vi "AlliGator Get Python Plugin Function Parameters String.vi"(8 "error in (no error)":errorcluster, 10 "Function Parameters":T1[](array[typedef]), 11 "Function Display Name":string) -> (0 "error out":errorcluster, 2 "Function Parameters JSON String":string, 3 "Parameter Names Not Found":string[](array[string]))   [LabVIEW 2021, in "AlliGator Python Plugins.lvlib"]
doc: "Gets requested parameter names from the python function description, opens up a dialog window to allow the user to enter the required parameters, and builds a JSON string to pass those parameters (names and values) to the python function."
uses:
  AlliGator Python Plugins.lvlib
  AlliGator Python Function Parameter Definition.ctl
  AlliGator Variables List.ctl
  d4008f8b-8ee3-446b-8e9c-2fee3dc7eda3.vi
  <userlib>/_OpenG.lib/string/string.llb/To Proper Case (String)__ogtk.vi
  <vilib>/JDP Science/JSONtext/Variant to JSON Text.vi
  <vilib>/JDP Science/JSONtext/support/Format JSON Object.vi
  <vilib>/JDP Science/JSONtext/LVClass Serializer/JSONtext LVClass Serializer.lvclass
  AlliGator Settings.lvlib
  AlliGator Globals, Variables & Constants.lvlib
  <vilib>/JDP Science/JSONtext/JSONtext.lvlib
  <userlib>/_OpenG.lib/string/string.llb/openg_string.lvlib
panel:
  # "see the AlliGator License on the block diagram (Ctrl+E or Window:Show Block Diagram)"
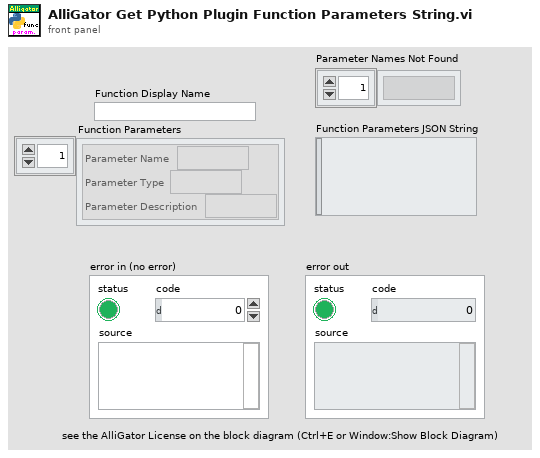
[diagram p1: front panel]
types:
  T1 = typedef "AlliGator Python Plugins.lvlib/AlliGator Python Function Parameter Definition.ctl" = cluster{"Parameter Name":string, "Parameter Type":string, "Parameter Description":string}
  T2 = typedef "AlliGator Globals, Variables & Constants.lvlib/AlliGator Variables List.ctl" = enum16{"---- GUI ----", "Initialization Status", "State Indicators Refnum", "Original AlliGator Menu Items", "Current Action Loop State", "Script in progress", "Playback", "Loop Playback", "Search ROI Used", "Search ROI", "Decay Graph Max Legend Size", "Intensity Graph Max Legend Size", "Decay Statistics Graph Max Legend Size", "Phasor Graph Max Legend Size", "Phasor Ratio Graph Max Legend Size", "Lifetime Graph Max Legend Size", "---- Files ----", "Export Dataset Frames as Individual Files", "Show Batch Export Help Balloons", "Frames in Dataset", "ptu File Frame Start Indices", "Current Frame in Dataset", "Current Frame Timestamp", "------ Python Plugins ------", "Python Plugins Information", "Python Session", "Valid Python Session?", "---- Source Image ----", "Dataset Loaded", "Dataset Metadata", "Dataset Channel", "Dataset Data Description", "Background Dataset Metadata", "Background Dataset Channel", "Background Dataset Data Description", "Background File Subtraction", "Background File Path", "Background File Pile-up Correction", "Background File Pixel Well Capacity", "Background File Scaling Factor", "Source Image ROIs", "Current Source Image ROI", "Source Image ROI Event Refnum", "X_Source Image Display Range", "X_Source Image Palette Information", "Source Image Palette List", "Source Image Scale", "Current Dataset Load Settings", "Source Image:ROI Overlay Color", "---- Image Profile Window ----", "Image Profile:Overlay ROI in Source Image", "Image Profile Window Event Refnum", "Image Profile:IntensityType", "Image Profile:Intensity Average Type", "Image Profile:Intensity-weighted SDV", "Image Profile:Box Profile Type", "Image Profile Window Open", "Image Profile:Plotted Fit Parameter", "X_Type of Displayed Image", "X_Time Gate Slider", "Dataset Path", "Source Image Overlay to Erase", "Is Displayed Image Accumulated", "White Light Image Modified", "Mask Image Modified", "Macrotime Gate Separation", "------ Phasor Graph -------", "Phasor Graph:Show Line", "---- Phasor Plot ---", "Phasor Plot Parameters Changed", "FLI Dataset Modified since last Phasor Plot Calculation", "Phasor Harmonics Data", "Selected Phasor Harmonics", "Phasor Harmonic Manager Event Refnum", "Phasor Plot ROIs", "Current Phasor Plot ROI", "Phasor Plot ROI Event Refnum", "Phasor Plot Image Reference Points", "Phasor Plot Computed", "Phasor Plot Palette Information", "Phasor Plot Palette List", "Phasor Ratio Palette Information", "Phasor Ratio Palette List", "Phasor Image Scale", "Phasor Plot Image Overlay to Erase", "Phasor Plot Image Elements to Update", "Current Phasor Plot Calculation Parameters", "Current Phasor Calibration Options", "Reset Cumulated Phasor Plot", "Phasor Ratio Reference 1", "Phasor Ratio Lifetime Reference 1", "Phasor Ratio Reference 1 Frequency", "Phasor Ratio Reference 2", "Phasor Ratio Lifetime Reference 2", "Phasor Ratio Reference 2 Frequency", "---- Decay Analysis ----", "Number of Selected Decays to Fit", "LS Fit Results", "LAR Fit Results", "BS Fit Results", "Last Decay Max - Min", "Best Fit Parameters", "Best Fit Parameter Names", "Actual Size X", "Actual Size Y", "Binning X", "Binning Y", "Actual # Gates", "Dataset Number", "Gates to...", "Gates Skipped", "Gates to keep", "Gate Step", "Gate Separation", "Reversed Gates", "Pile-up Correction", "Pixel Well Capacity", "Background Subtracted", "Background Subtraction Method", "Background Definition Range", "Background File (deprecated)", "Number of Dataset Accumulated", "Array of Accumulated Dataset Paths", "Do Averaged Datasets", "Destination File Path", "Process Plot Target", "Use 1/D as Phasor Frequency", "---- Decay Fit Parameter Map -----", "Decay Fit Parameter Map Palette Information", "Decay Fit Parameter Map Palette List", "Local Decay Graph Window Event Refnum", "------- Local Decay Window ---------", "Use normalized IRF for convolution", "----- Miscellaneous ----", "Skippable Dialog Windows Status"}
  T3 = typedef "AlliGator Settings.lvlib/AlliGator Settings List.ctl" = enum16{"GUI:Visible Settings Tab", "GUI:Last Run Version", "Source Image:Use Image Histogram for Contrast", "Source Image:Low Count Pixels Rejection Options", "Source Image:High Count Pixels Rejection Options", "Source Image:Use Image Brightness", "Source Image:Blend Overlay with Image Background", "Source Image:Use Fixed ROI Diameter", "Source Image:ROI Diameter", "Source Image:ROI Center Color", "Source Image:Peak Threshold", "Source Image:Intensity Threshold", "Source Image:Image Binning Options", "Source Image:Image Smoothing Options", "Source Image:Image Histogram Active", "Source Image:Invert Binary Mask", "Source Image:Hot Pixel Removal", "Source Image:Overlay Analyzed ROI Center", "Source Image:Auto-Adjust Contrast", "Source Image:Histogram Lower Percentile", "Source Image:Histogram Upper Percentile", "Source Image:Save Source Image", "Source Image:Scale Bar Options", "Source Image:Image Resolution (Pixel Size)", "Source Image:Flatfield Correction", "Data Information:Gate Width", "Data Information:Nanotime Gate Separation", "Data Information:Macrotime Gate Separation", "Data Information:Gate Step", "Data Information:# Gates", "Data Information:Gate Image Exposure", "Data Information:Gate Image Integration", "Data Information:Gates to Skip", "Data Information:Gates to Keep", "Data Information:Define Gates to", "Data Information:Channel Name", "Data Information:Available Channel Names", "Data Information:Channel Arithmetic", "Data Information:Background File Subtraction", "Data Information:Background File", "Data Information:Background Scaling Factor", "Data Information:Background Pile-up Correction", "Data Information:Background Pixel Well Capacity", "Data Information:Laser Period", "Data Information:SYNC Period", "Data Information:Pile-up Correction", "Data Information:Pixel Well Capacity", "Data Information:Dataset Scaling Factor", "Fluorescence Decay_Decay Pre-Processing:Reverse Gates", "Fluorescence Decay_Decay Pre-Processing:Verbose Decay Pre-Processing", "Fluorescence Decay_Decay Pre-Processing:Use Decay Pre-Processing", "Fluorescence Decay_Decay Pre-Processing:Background Subtraction", "Fluorescence Decay_Decay Pre-Processing:Background Definition Range", "Fluorescence Decay_Decay Pre-Processing:Baseline Subtraction Method", "Fluorescence Decay_Decay Pre-Processing:Operations Order", "Fluorescence Decay_Decay Pre-Processing:Smoothing Parameter", "Fluorescence Decay_Decay Pre-Processing:Shift Decay", "Fluorescence Decay_Decay Pre-Processing:Decay Shift Parameters", "Fluorescence Decay_Decay Pre-Processing:Fold Decay", "Fluorescence Decay_Decay Pre-Processing:# Folds", "Fluorescence Decay_Decay Pre-Processing:1-Normalize Decay", "Fluorescence Decay_Decay Pre-Processing:[0-1]-Normalize Decay", "Fluorescence Decay_Decay Pre-Processing:Smoothen Decay", "Fluorescence Decay_Decay Pre-Processing:Extrapolate Decay", "Fluorescence Decay_Decay Pre-Processing:Use Periodicity", "Fluorescence Decay_Decay Pre-Processing:Use Cursors", "Fluorescence Decay_Decay Pre-Processing:Tail Fraction", "Fluorescence Decay_Decay Pre-Processing:Head Fraction", "Fluorescence Decay_Decay Pre-Processing:Additional Points", "Fluorescence Decay_Decay Pre-Processing:Straighten Decay", "Fluorescence Decay_Decay Pre-Processing:Constant Background", "Fluorescence Decay_Decay Pre-Processing:Pixel-Normalize Decay", "Fluorescence Decay_Advanced Analysis:Extract IRF instead of Decay", "Fluorescence Decay_Advanced Analysis:IRF Extraction Options", "Fluorescence Decay_Advanced Analysis:IRF Optimization Options", "Fluorescence Decay_Advanced Analysis:Square Pulse Options", "Fluorescence Decay_Advanced Analysis:IRF Order", "Fluorescence Decay_Advanced Analysis:IRF Time Constants", "Fluorescence Decay_Advanced Analysis:Wavelet Analysis Options", "Fluorescence Decay_Advanced Analysis:Average Lifetime Options", "Fluorescence Decay_Fit Options:Fit Options", "Fluorescence Decay_Fit Options:Use Legacy Fitting Approach", "Fluorescence Decay_Fit Options:Use Data Information Laser Period", "Fluorescence Decay_Fit Parameters:Displayed Fit Parameters", "Fluorescence Decay_Fit Parameters:Fit Parameter Constraints", "Fluorescence Decay_Fit Parameters:Export Tabulated Results", "Fluorescence Decay_Fit Parameters:MLE Baseline Offset Type", "Fluorescence Decay_Fit Parameters:MLE Baseline Offset", "Fluorescence Decay_Fit Parameters:Guess Parameter Names", "Fluorescence Decay_Fit Parameters:Guess Parameter Values", "Fluorescence Decay_Fit Parameters:Guess Parameters Options", "Fluorescence Decay_Styles:Show Last Decay Only", "Fluorescence Decay_Styles:Decay Graph Color Array", "Fluorescence Decay:Decay Graph Active", "Fluorescence Decay Statistics:Min Peak Value", "Fluorescence Decay Statistics:Reject Low Decay Peak Pixels", "Fluorescence Decay Statistics:Reject High Decay Peak Pixels", "Fluorescence Decay Statistics:Max Peak Value", "Time Traces:Use File Timestamp", "Time Traces:Time Step", "Time Traces:Use Intensity Correction File", "Time Traces:Intensity Correction File", "Phasor Plot:Phasor Plot Smoothing Options", "Phasor Plot:Phasor Plot Size", "Phasor Plot:Phasor Plot Graphics Options", "Phasor Plot:Cumulative Phasor Plot", "Phasor Plot:Use Phasor Brightness", "Phasor Plot:Blend Overlay with Phasor Background", "Phasor Plot:Save Phasor Plot", "Phasor Plot:Show References", "Phasor Plot:Phasor Ratio Decay Range", "Phasor Plot:Exponential Fading", "Phasor Plot:Phasor Ratio Reference Colors", "Phasor Plot:Reference Radius", "Phasor Plot:Show Color Map Vertices", "Phasor Plot:Phasor Plot Active", "Phasor Plot:Phasor Ratio Color Map Type", "Phasor Plot:Phasor Ratio Color Map", "Phasor Plot:Phasor Ratio Display Range", "Phasor Plot:Selected Image ROI(s)", "Phasor Plot:All Image ROIs", "Phasor Plot:Selected Phasor Plot ROI(s)", "Phasor Plot:All Phasor Plot ROIs", "Phasor Plot:Phasor Ratio Color-Coded Quantity", "Phasor Plot:Store Phasor Harmonics", "Phasor Plot:Draw Reference Segment", "Phasor Plot:User-Defined Quantity", "Phasor Graph:Phasor Frequency", "Phasor Graph:Phasor Ratio Type", "Phasor Graph:Pixel-level Phasor Computation", "Phasor Graph:Save Phasor Graph", "Phasor Graph:Phasor Graph Active", "Phasor Graph:Phasor SDV Options", "Phasor Calibration:Use Backup Calibration if needed", "Phasor Graph:Define Shortest Lifetime as", "Phasor Calibration:Backup Calibration Type", "Phasor Calibration:Calibration Type", "Phasor Calibration:Calibration Lifetime", "Phasor Calibration:Calibration Map Algorithm", "Single-Exponential Phasor Locus (SEPL):Gate Parameters", "Single-Exponential Phasor Locus (SEPL):User-defined Gate", "Single-Exponential Phasor Locus (SEPL):User-defined IRF", "Single-Exponential Phasor Locus (SEPL):Phasor Parameters", "Single-Exponential Phasor Locus (SEPL):Decay & IRF Parameters", "Single-Exponential Phasor Locus (SEPL):Display Parameters", "Lifetime Analysis:Decay Analysis Parameters", "Lifetime Analysis:Lifetime Map Active", "Plugins:Python Settings", "Miscellaneous:Verbose Mode", "Miscellaneous:Beep after Script", "Miscellaneous:Saved Image File Format", "Miscellaneous:Exported Gate Image Settings", "Miscellaneous:Include Loading in Timing", "Miscellaneous:Verbose Settings Mode", "Miscellaneous:Histogram Options", "Miscellaneous:Beep on Error", "Miscellaneous:# Logical Processors Used", "Miscellaneous:ROI Description Max Characters", "Miscellaneous:Verbose Error Mode", "Miscellaneous:Transparent Mask Color"}
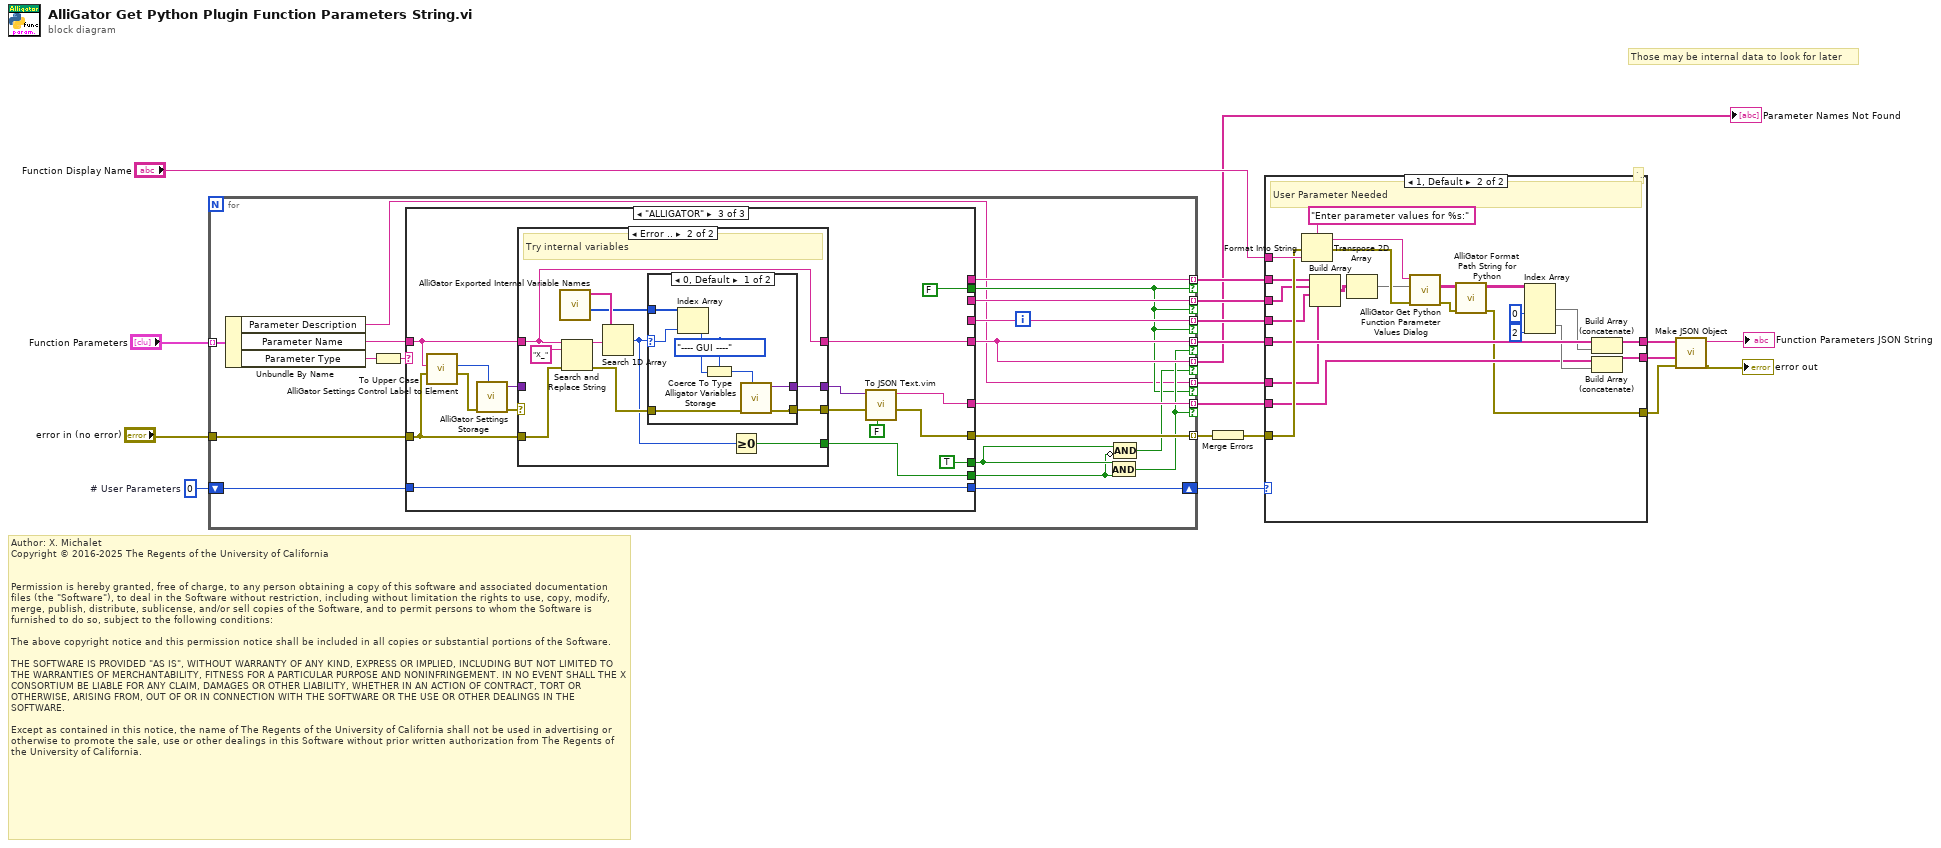
[diagram p0: block diagram]
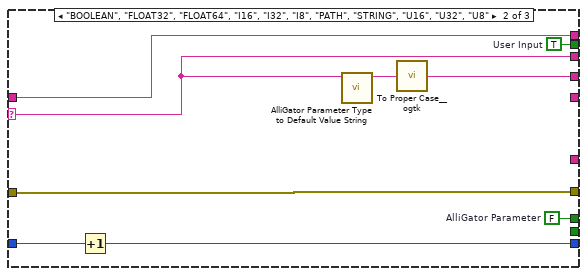
[diagram p4: hidden frame]
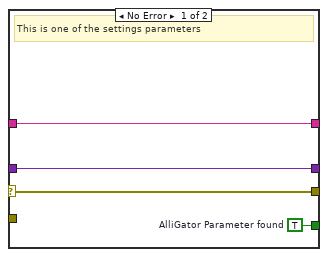
[diagram p5: hidden frame]
diagram:
  w14 = 0  # # User Parameters
  # "Author: X. Michalet\nCopyright © 2016-2025 The Regents of the University of California\n \n\nPermission is hereby granted, free of charge, to any person obtaining a copy of this software and associated documentation files (the \"Software\"), to deal in the Software without restriction, including without limitation the rights to use, copy, modify, merge, publish, distribute, sublicense, and/or sell copies of the Software, and to permit persons to whom the Software is furnished to do so, subject to the following conditions:\n\nThe above copyright notice and this permission notice shall be included in all copies or substantial portions of the Software.\n\nTHE SOFTWARE IS PROVIDED \"AS IS\", WITHOUT WARRANTY OF ANY KIND, EXPRESS OR IMPLIED, INCLUDING BUT NOT LIMITED TO THE WARRANTIES OF MERCHANTABILITY, FITNESS FOR A PARTICULAR PURPOSE AND NONINFRINGEMENT. IN NO EVENT SHALL THE X CONSORTIUM BE LIABLE FOR ANY CLAIM, DAMAGES OR OTHER LIABILITY, WHETHER IN AN ACTION OF CONTRACT, TORT OR OTHERWISE, ARISING FROM, OUT OF OR IN CONNECTION WITH THE SOFTWARE OR THE USE OR OTHER DEALINGS IN THE SOFTWARE.\n\nExcept as contained in this notice, the name of The Regents of the University of California shall not be used in advertising or otherwise to promote the sale, use or other dealings in this Software without prior written authorization from The Regents of the University of California."
  # "``"
  # "Those may be internal data to look for later"
  n1 = for {
    tunnel: "Function Parameters" -> [w38] mode=indexing
    tunnel: [w35] -> w18 mode=indexing
    tunnel: "error in (no error)" -> [w34]
    shift-right: [w32] -> w13
    shift-left: w14 -> [w33]
    tunnel: [w31] -> w12 mode=indexing if=w25
    tunnel: [w27] -> w11 mode=indexing if=w25
    tunnel: [w30] -> w10 mode=indexing if=w21
    tunnel: [w29] -> w9 mode=indexing if=w21
    tunnel: [w28] -> w8 mode=indexing if=w21
    tunnel: [w27] -> w2 mode=indexing if=w22
    tunnel: [w20] -> w1 mode=indexing if=w21
    n2 = Unbundle By Name(w38) -> ("Parameter Description"=w20:string, "Parameter Name"=w37:string, "Parameter Type"=w36:string)
    n3 = To Upper Case(1:w36) -> (0:w26:string)
    n4 = case shown="\"ALLIGATOR\"" w26 {
      selector: w26 -> [_ w44 _]
      tunnel: w37 -> [_ w47 w55]
      tunnel: [w40 w46 w50] -> w35
      tunnel: w34 -> [w40 w46 w57]
      tunnel: w33 -> [w39 w49 w63]
      tunnel: [w39 w48 w63] -> w32
      tunnel: [_ _ w56] -> w31
      tunnel: [_ _ w54] -> w27
      tunnel: [_ w42 TRUE ("AlliGator Parameter")] -> w24
      tunnel: [_ w47 _] -> w30
      tunnel: [_ w44 _] -> w29
      tunnel: [_ w45 FALSE ("Pretty Print?")] -> w21
      tunnel: [_ w41 _] -> w28
      tunnel: [_ _ w51] -> w23
      frame "", Default {
      }
      frame "BOOLEAN", "FLOAT32", "FLOAT64", "I16", "I32", "I8", "PATH", "STRING", "U16", "U32", "U8" {
        w42 = FALSE  # AlliGator Parameter
        w45 = TRUE  # User Input
        n5 = Increment(x=w49) -> (x+1=w48:i32)
        n6 = call "AlliGator Parameter Type to Default Value String.vi"("Parameter Type"=w44) -> ("Default Parameter String"=w43:string)  [unwired: 10 in]
        n7 = call-poly <userlib>:"To Proper Case__ogtk.vi"("string"=w43) -> ("proper case string"=w41:string)  [unwired: 4 in]
      }
      frame "ALLIGATOR" {
        n8 = call "AlliGator Settings Control Label to Element.vi"("Error In"=w57, "Control Label"=w55) -> ("Error Out"=w62:errorcluster, "AlliGator Settings List Element"=w65:T3)  [unwired: 6 in]
        n9 = call "AlliGator Settings Storage.vi"("AlliGator Settings List"=w65, "Error In"=w62) -> ("Error Out"=w61:errorcluster, "Variant Data out"=w60:variant)  [unwired: 8 in]
        n10 = case shown="Error .." w61 {
          selector: w61 -> [w69 _]
          tunnel: w60 -> [w68 _]
          tunnel: [w69 w80] -> w59
          tunnel: [w68 w79] -> w58
          tunnel: w57 -> [_ w77]
          tunnel: w55 -> [w67 w72]
          tunnel: [w67 w72] -> w54
          tunnel: [w66 w70] -> w51
          frame No Error {
            w66 = TRUE  # AlliGator Parameter found
            # "This is one of the settings parameters"
          }
          frame Error {
            # "Try internal variables"
            n11 = call "AlliGator Exported Internal Variable Names.vi"() -> ("Indices of Exported IVs"=w74:i32[], "Exported IV Name Array"=w76:string[])  [unwired: 10 in]
            n12 = Search and Replace String(input string=w72, search string="X_" ("replace string (\"\")"), error in=w77) -> (result string=w75:string, error out=w78:errorcluster)  [unwired: 5 in, 2 out]
            n13 = Search 1D Array(1D array=w76, element=w75) -> (index of element=w71:i32)  [unwired: 1 in]
            n14 = case shown="0, Default" w71 {
              selector: w71 -> [w82 _]
              tunnel: [w88 w89] -> w80
              tunnel: [w87 _] -> w79
              tunnel: w78 -> [w84 w89]
              tunnel: w74 -> [w83 _]
              frame 0, Default {
                n15 = Index Array(array=w83, index=w82) -> (element=w81:i32)
                n16 = Coerce To Type(0:w81, 1:AlliGator_Variables_List."---- GUI ----" ("Alligator Variable")) -> (2:w86:T2)
                n17 = call "Alligator Variables Storage.vi"("AlliGator Variable"=w86, "Error In"=w84) -> ("Error Out"=w88:errorcluster, "Data out"=w87:variant)  [unwired: 7 in, 1 out]
              }
              frame -1 {
                # "not found"
              }
            }
            n18 = Greater Or Equal To 0?(x=w71) -> (x >= 0?=w70:bool)
          }
        }
        n19 = call "To JSON Text.vim"("Pretty Print?"=FALSE, "error in (no error)"=w59, "Anything"=w58) -> ("error out"=w50:errorcluster, "<JSON>"=w56:string)  [unwired: 7 in]
      }
    }
    n20 = And(x=w24, y=w23) -> (x .and. y?=w25:bool)
    n21 = Compound Arithmetic op=AND(w24, invert w23) -> (w22:bool)
  }
  "Parameter Names Not Found" <- w2
  n22 = Merge Errors(w18) -> (w16:errorcluster)
  n23 = case shown="1, Default" w13 {
    tunnel: "Function Display Name" -> [_ w115]
    tunnel: [w92 w94] -> w7
    tunnel: w16 -> [w92 w111]
    tunnel: w12 -> [w91 w101]
    tunnel: w11 -> [w90 w105]
    tunnel: w10 -> [_ w110]
    tunnel: w9 -> [_ w109]
    tunnel: w8 -> [_ w108]
    tunnel: [w91 w100] -> w5
    tunnel: [w90 w103] -> w4
    tunnel: w1 -> [_ w93]
    frame 0 {
      # "No user-input needed"
    }
    frame 1, Default {
      # "User Parameter Needed"
      n24 = Format Into String(format string="Enter parameter values for %s:", error in=w111, w115) -> (resulting string=w113:string, error out=w112:errorcluster)  [unwired: 1 in]
      n25 = Build Array(w110, w109, w108, w93) -> (w107:string[][])
      n26 = Transpose 2D Array(2D array=w107) -> (transposed array=w97:string[][])
      n27 = call "AlliGator Get Python Function Parameter Values Dialog.vi"("Error In"=w112, "Parameters In"=w97, "Input Message"=w113) -> ("Error Out"=w95:errorcluster, "Parameters Out"=w106:string[][])  [unwired: 6 in, 1 out]
      n28 = call "AlliGator Format Path String for Python.vi"("Error In"=w95, "Python Plugin Dialog Output"=w106) -> ("Error Out"=w94:errorcluster, "Python Plugin Dialog Output"=w96:string[][])  [unwired: 8 in]
      n29 = Index Array(array=w96, index (col) #1=0 ("disabled index (col)"), index (col) #2=2 ("index (col)")) -> (element #1=w104:string[], element #2=w102:string[])  [unwired: 2 in]
      n30 = Build Array (concatenate)(w105, w104) -> (w103:string[])
      n31 = Build Array (concatenate)(w101, w102) -> (w100:string[])
    }
  }
  n32 = call <vilib>:"Make JSON Object.vi"("error in (no error)"=w7, "JSON Items"=w5, "Item Names"=w4) -> ("error out"=→"error out":errorcluster, "<JSON>"=→"Function Parameters JSON String":string)  [unwired: 7 in]
